vi "Results search.vi"(11 "Results":string[][](array[string])) -> (3 "p/f":bool)   [LabVIEW 2012]
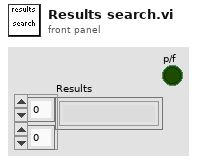
[diagram p1: front panel]
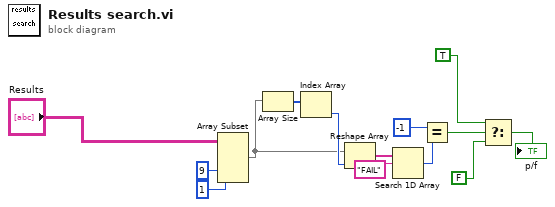
[diagram p0: block diagram]
diagram:
  n1 = Array Subset(array="Results", index (col)=9 ("index"), length (col)=1 ("length")) -> (w6:string[][])  [unwired: 2 in]
  n2 = Array Size(array=w6) -> (size(s)=w7:i32[])
  n3 = Index Array(array=w7) -> (element=w8:i32)  [unwired: 1 in]
  n4 = Reshape Array(w6, w8) -> (w9:string[])
  n5 = Search 1D Array(1D array=w9, element="FAIL") -> (index of element=w11:i32)  [unwired: 1 in]
  n6 = Equal?(x=-1, y=w11) -> (x = y?=w13:bool)
  n7 = Select(t=TRUE, s=w13, f=FALSE) -> (s? t:f=→"p/f":bool)
